vi "Set Wavelength Status Broadcast.vi"(8 "error in":errorcluster, 10 "Reply Payload":T1) -> (0 "error out":errorcluster)   [LabVIEW 2020, in "Topas.lvlib"]
doc: "Get the status of the wavelength change.\n_____\nCreated using DQMH Event Scripter 6.0.0.122."
uses:
  Topas.lvlib
  Get Wavelength Set Status (Reply Payload)--cluster.ctl
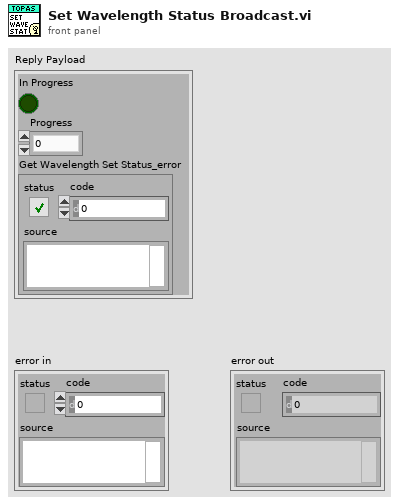
[diagram p1: front panel]
types:
  T1 = typedef "Topas.lvlib/Get Wavelength Set Status (Reply Payload)--cluster.ctl" = cluster{"In Progress":bool, "Progress":dbl, "Get Wavelength Set Status_error":errorcluster}
  T2 = typedef "Topas.lvlib/Broadcast Events--cluster.ctl" = cluster{"Module Did Init":refnum<user-event>, "Status Updated":refnum<user-event>, "Error Reported":refnum<user-event>, "Module Did Stop":refnum<user-event>, "Update Module Execution Status":refnum<user-event>, "Broadcast Topas Wavelength":refnum<user-event>, "Set Wavelength Status Broadcast":refnum<user-event>}
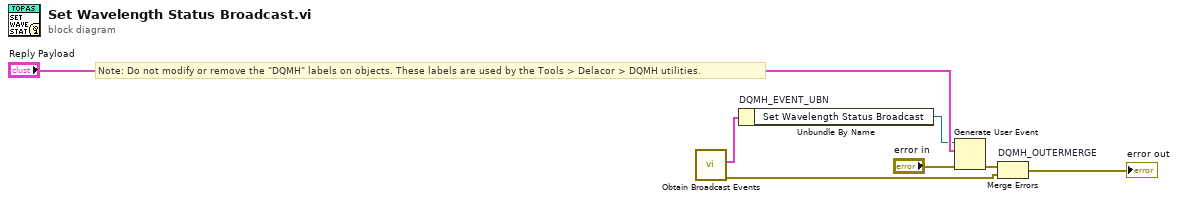
[diagram p0: block diagram]
diagram:
  # "Note: Do not modify or remove the \"DQMH\" labels on objects. These labels are used by the Tools > Delacor > DQMH utilities."
  n1 = call "Obtain Broadcast Events.vi"() -> ("error out"=w2:errorcluster, "Topas Broadcast Events"=w1:T2)  [unwired: 10 in]
  n2 = Unbundle By Name "DQMH_EVENT_UBN"(w1) -> ("Set Wavelength Status Broadcast"=w4:refnum<user-event>)
  n3 = Generate User Event(user event=w4, event data cluster="Reply Payload", error in="error in") -> (error out=w3:errorcluster)  [unwired: 1 in, 1 out]
  n4 = Merge Errors "DQMH_OUTERMERGE"(w3, w2) -> (→"error out":errorcluster)
